vi "fgv_scout_data.vi"(7 "cmd":enum16{"write", "read"}(ring), 11 "raw data":string) -> (3 "agv data out":T1)   [LabVIEW 2019]
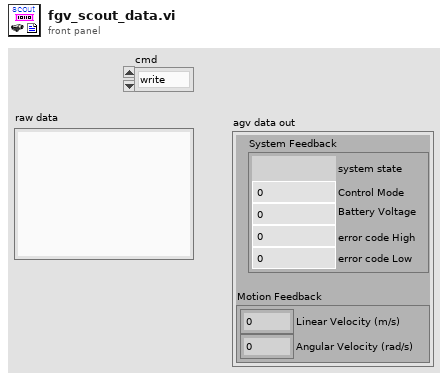
[diagram p1: front panel]
types:
  T1 = cluster{"System Feedback":cluster{"system state":string, "Control Mode":u8, "Battery Voltage":dbl, "error code High":u8, "error code Low":u8}, "Motion Feedback":cluster{"Linear Velocity (m/s)":dbl, "Angular Velocity (rad/s)":dbl}}
  T2 = cluster{"system state":string, "Control Mode":u8, "Battery Voltage (V)":dbl, "error code High":u8, "error code Low":u8}
  T3 = cluster{"Linear Velocity (m/s)":dbl, "Angular Velocity (rad/s)":dbl}
  T4 = cluster{"System Feedback":cluster{"system state":string, "Control Mode":u8, "Battery Voltage (V)":dbl, "error code High":u8, "error code Low":u8}, "Motion Feedback":cluster{"Linear Velocity (m/s)":dbl, "Angular Velocity (rad/s)":dbl}}
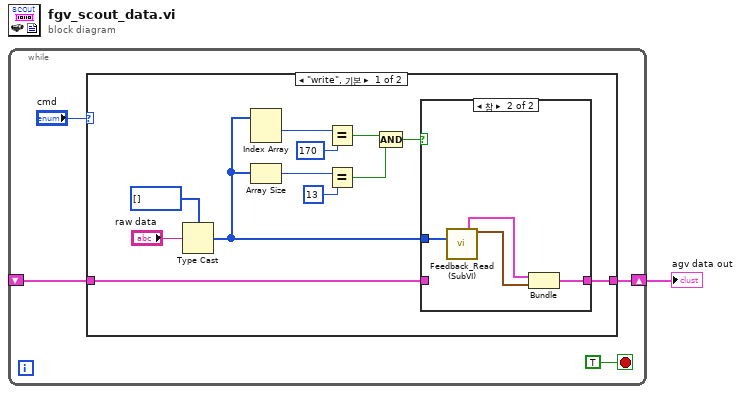
[diagram p0: block diagram]
diagram:
  n1 = while {
    shift-right: [w3] -> w1
    shift-left: _ -> [w2]
    stop <- TRUE stop-if-true
    n2 = case shown="\"write\", 기본" "cmd" {
      tunnel: [w7 w23] -> w3
      tunnel: w2 -> [w6 w23]
      frame "write", Default {
        n3 = Type Cast(type=i8[] [], x="raw data") -> (*(type *) &x=w8:i8[])
        n4 = Index Array(array=w8) -> (element #1=w11:i8)  [unwired: 2 in, 1 out]
        n5 = Array Size(array=w8) -> (size(s)=w13:i32)
        n6 = Equal?(x=w11, y=u8 170) -> (x = y?=w15:bool)
        n7 = Equal?(x=w13, y=13) -> (x = y?=w16:bool)
        n8 = Compound Arithmetic op=AND(w15, w16) -> (w9:bool)
        n9 = case shown="참" w9 {
          tunnel: w8 -> [_ w22]
          tunnel: [w18 w20] -> w7
          tunnel: w6 -> [w18 _]
          frame False {
          }
          frame True {
            n10 = call "Feedback_Read (SubVI).vi"("System State Feedback"=w22) -> ("System Feedback"=w19:T2, "Motion Feedback"=w21:T3)  [unwired: 7 in, 6 out]
            n11 = Bundle("System Feedback"=w19, "Motion Feedback"=w21) -> (w20:T4)  [unwired: 1 in]
          }
        }
      }
      frame "read" {
      }
    }
  }
  "agv data out" <- w1
